vi "Handle Error.vi"(8 "error in (no error)":errorcluster, 11 "Post Analysis in":refnum<class "Post Analysis.lvclass">) -> (0 "error out":errorcluster, 2 "stop actor?":bool=TRUE, 3 "Post Analysis out":refnum<class "Post Analysis.lvclass">)   [LabVIEW 2023, in "Data Analysis.lvlib" / "Post Analysis.lvlib" / "Post Analysis.lvclass"]
doc: "(<B>Filename</B>: Actor Framework.lvlib:Actor.lvclass:Handle Error.vi)\n\nDefines how the actor handles an error that occurred while processing a message. By default, this method does nothing except stop the actor."
uses:
  Post Analysis.lvclass
  <vilib>/Utility/error.llb/DialogType.ctl
  <vilib>/ActorFramework/Actor/Actor.lvclass
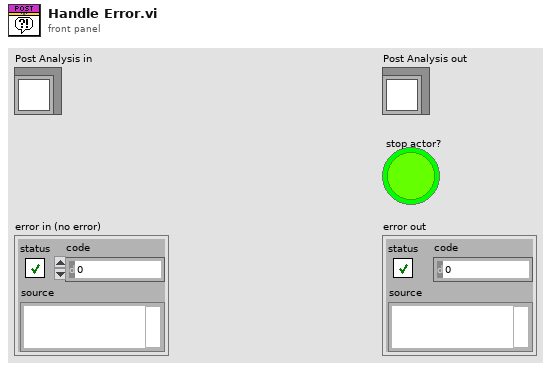
[diagram p1: front panel]
types:
  T1 = typedef "DialogType.ctl" = u16
  T2 = enum16{"Open", "Read File", "Write File", "Close"}
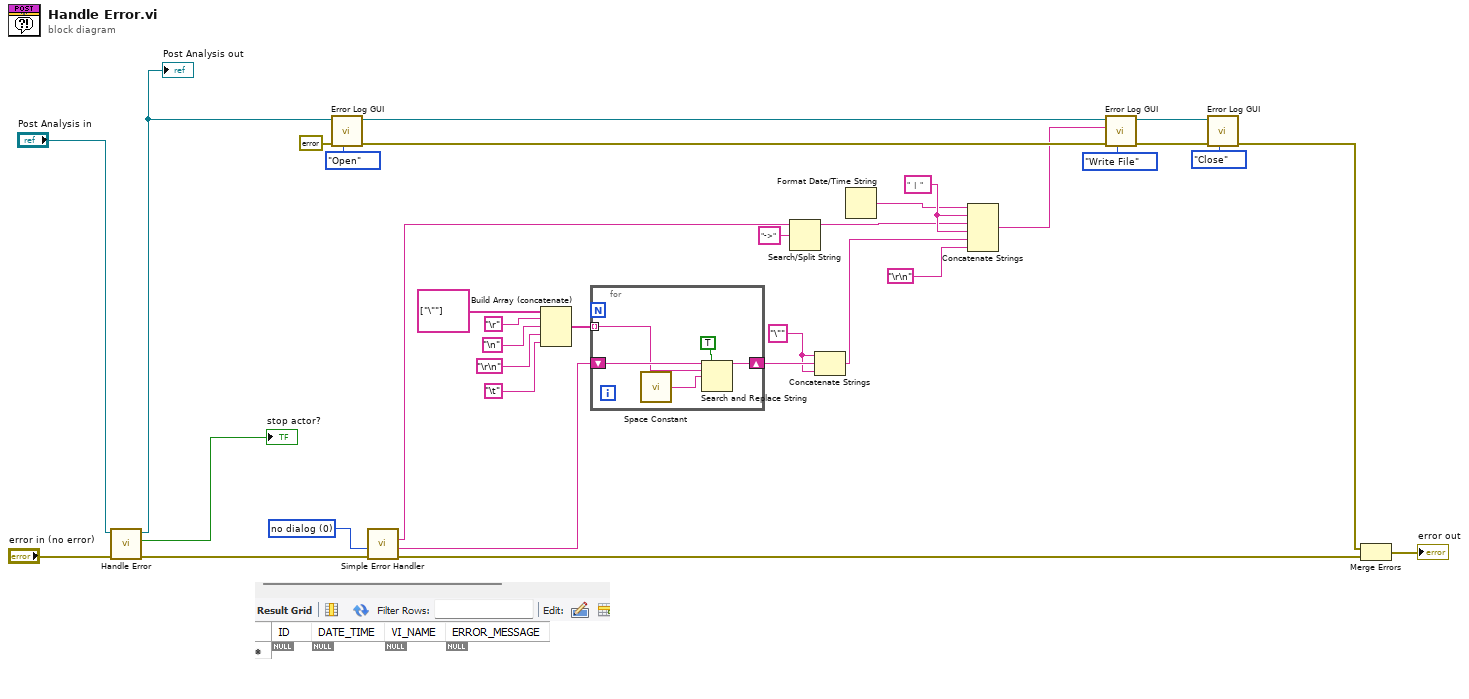
[diagram p0: block diagram]
diagram:
  w9 = "\"" ("string")
  w12 = "  |  "
  w14 = T1 0 items=["no dialog", "OK message", "continue or stop message", "OK message + warnings", "continue/stop + warnings"] ("type of dialog (OK msg:1)")
  n1 = call-parent "Handle Error.vi"("error in (no error)"="error in (no error)", "Actor in"="Post Analysis in") -> ("error out"=w31:errorcluster, "stop actor?"=→"stop actor?":bool, "Actor out"=w26:refnum<class "Post Analysis.lvclass">)  [unwired: 7 in]
  "Post Analysis out" <- w26
  n2 = call "Error Log GUI.vi"("File Options"=T2."Open", "error in (no error)"=errorcluster {"status"=FALSE, "code"=0, "source"=""}, "Post Analysis in"=w26) -> ("error out"=w24:errorcluster, "Post Analysis out"=w25:refnum<class "Post Analysis.lvclass">)  [unwired: 7 in]
  n3 = call <vilib>:"Simple Error Handler.vi"("type of dialog (OK msg:1)"=w14, "error in (no error)"=w31) -> ("source out"=w13:string, "error out"=w15:errorcluster, "message"=w5:string)  [unwired: 3 in, 2 out]
  n4 = Build Array (concatenate)(string[] ["\""], "\r", "\n", "\r\n", "\t") -> (w21:string[])
  n5 = for {
    tunnel: w21 -> [w36] mode=indexing
    shift-right: [w37] -> w10
    shift-left: w13 -> [w38]
    n6 = call <vilib>:"Space Constant.vi"() -> ("String"=w35:string)
    n7 = Search and Replace String(replace all?=TRUE ("replace all? (F)"), input string=w38, search string=w36, replace string=w35) -> (result string=w37:string)  [unwired: 4 in, 3 out]
  }
  n8 = Search/Split String(string=w5, search string/char (-)="->") -> (substring before match=w4:string)  [unwired: 1 in, 2 out]
  n9 = Concatenate Strings(w9, w10, w9) -> (w8:string)
  n10 = Format Date/Time String() -> (date/time string=w11:string)  [unwired: 3 in]
  n11 = Concatenate Strings(w11, w12, w4, w12, w8, "\r\n") -> (w6:string)
  n12 = call "Error Log GUI.vi"("File Options"=T2."Write File", "error in (no error)"=w24, "Write"=w6, "Post Analysis in"=w25) -> ("error out"=w28:errorcluster, "Post Analysis out"=w29:refnum<class "Post Analysis.lvclass">)  [unwired: 6 in]
  n13 = call "Error Log GUI.vi"("File Options"=T2."Close", "error in (no error)"=w28, "Post Analysis in"=w29) -> ("error out"=w2:errorcluster)  [unwired: 7 in, 1 out]
  n14 = Merge Errors(w2, w15) -> (→"error out":errorcluster)
